vi "test.ingest_containerized.vi"   [LabVIEW 2020]
uses:
  datasources/dataset/dataset.lvclass
  81c5314d-0c17-4e40-9591-806fc92e59be.vi
  Nominal Client/Nominal Client.lvclass
  40e2c779-94f0-4ff6-913c-6196809b7e71.vi
  datasources/source/source.lvclass
  datasources/target/target.lvclass
  nominal types/channelConfig/channelConfig.lvclass
  Nominal Client/ingest_containerized.vi
  datasources/source/create_s3.vi
  datasources/source/create_gcs.vi
  datasources/target/create_from_existing.vi
  datasources/target/create_new.vi
  nominal types/properties/properties.lvclass
  datasources/gcs/gcs.lvclass
  C:/code/labview-client/lv_src/Nominal Client/datasources/source/source.lvclass
  C:/code/labview-client/lv_src/Nominal Client/datasources/payload/payload.lvclass
  C:/code/labview-client/lv_src/Nominal Client/datasources/gcs/gcs.lvclass
  datasources/s3/s3.lvclass
  C:/code/labview-client/lv_src/Nominal Client/datasources/s3/s3.lvclass
types:
  T1 = cluster{"dataset":refnum<class "dataset.lvclass">, "channelConfig":refnum<class "channelConfig.lvclass">}
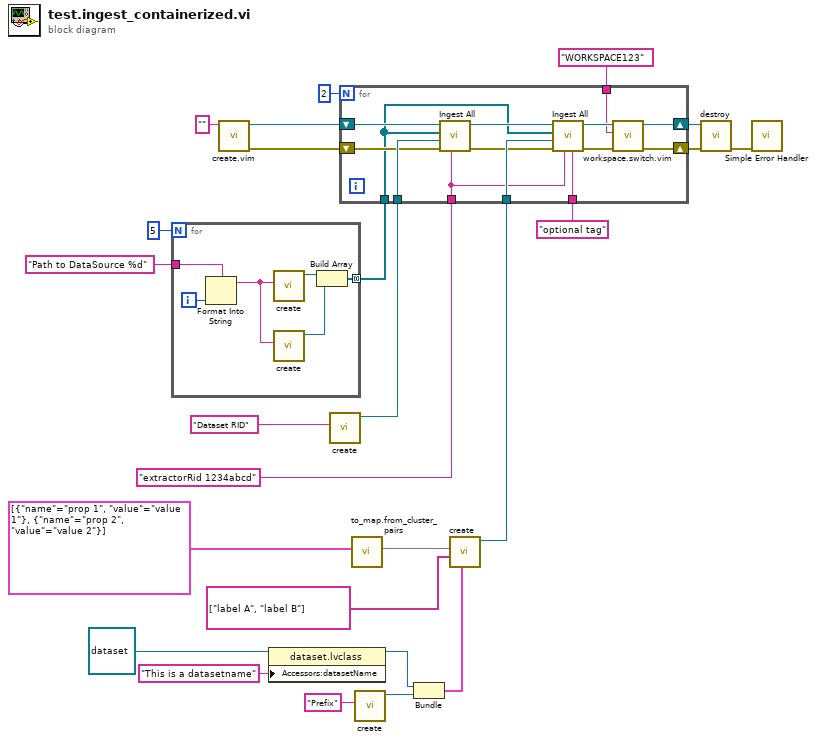
[diagram p0: block diagram]
diagram:
  n1 = for {
    N: 5 -> [_]
    tunnel: "Path to DataSource %d" ("Path") -> [w30]
    tunnel: [w26] -> w7 mode=concatenating
    i -> [w29]
    n2 = Format Into String(format string=w30, w29) -> (resulting string=w31:string)  [unwired: 2 in, 1 out]
    n3 = call-poly "create.vi"("Path"=w31) -> ("source"=w28:refnum<class "gcs.lvclass">)  [unwired: 10 in]
    n4 = call-poly "create.vi"("Path"=w31) -> ("source"=w27:refnum<class "s3.lvclass">)  [unwired: 10 in]
    n5 = Build Array(w28, w27) -> (w26:refnum<class "source.lvclass">[])
  }
  n6 = call "create.vim"("API Token (string or path)"="") -> ("error out"=w21:errorcluster, "Nominal Client"=w22:refnum<class "Nominal Client.lvclass">)  [unwired: 9 in]
  n7 = property class="dataset.lvclass"(reference=refnum<class "dataset.lvclass"> refnum ("dataset"), "Accessors:datasetName"="This is a datasetname" ("datasetName")) -> (reference out=w17:refnum<class "dataset.lvclass">)  [unwired: 1 in, 1 out]
  n8 = call-poly "create.vi"("dataset RID"="Dataset RID" ("RID")) -> ("Existing Target"=w14:refnum<class "target.lvclass">)  [unwired: 10 in]
  n9 = call "to_map.from_cluster_pairs.vi"("properties (cluster pairs)"=cluster{"name":string, "value":string}[] [{"name"="prop 1", "value"="value 1"}, {"name"="prop 2", "value"="value 2"}] ("properties")) -> ("properties (map)"=w1:map{string, string})  [unwired: 10 in]
  n10 = call "create.vi"("prefixTreeDelimiter"="Prefix") -> ("channelConfig"=w10:refnum<class "channelConfig.lvclass">)  [unwired: 10 in]
  n11 = Bundle("dataset"=w17, "channelConfig"=w10) -> (w13:T1)  [unwired: 1 in]
  n12 = call-poly "create.vi"("Optional"=w13, "Labels"=string[] ["label A", "label B"] ("labels"), "Properties"=w1) -> ("New Target"=w12:refnum<class "target.lvclass">)  [unwired: 8 in]
  n13 = for {
    N: 2 -> [_]
    tunnel: w14 -> [w45]
    tunnel: w7 -> [w34]
    tunnel: w12 -> [w44]
    shift-right: [w37] -> w23
    shift-left: w21 -> [w41]
    shift-right: [w36] -> w25
    shift-left: w22 -> [w40]
    tunnel: "WORKSPACE123" ("RID") -> [w35]
    tunnel: "extractorRid 1234abcd" ("RID") -> [w33]
    tunnel: "optional tag" ("RID") -> [w32]
    n14 = call-poly "Ingest All.vi"("extractorRid"=w33, "error in"=w41, "Target"=w45, "sources"=w34, "Nominal Client in"=w40) -> ("error out"=w42:errorcluster, "Nominal Client out"=w43:refnum<class "Nominal Client.lvclass">)  [unwired: 3 in, 2 out]
    n15 = call-poly "Ingest All.vi"("tag"=w32, "extractorRid"=w33, "error in"=w42, "Target"=w44, "sources"=w34, "Nominal Client in"=w43) -> ("error out"=w38:errorcluster, "Nominal Client out"=w39:refnum<class "Nominal Client.lvclass">)  [unwired: 2 in, 2 out]
    n16 = call "workspace.switch.vim"("error in"=w38, "Workspace RID (string or path)"=w35, "Nominal Client in"=w39) -> ("error out"=w37:errorcluster, "Nominal Client out"=w36:refnum<class "Nominal Client.lvclass">)  [unwired: 7 in]
  }
  n17 = call "destroy.vi"("error in"=w23, "Nominal Client"=w25) -> ("error out"=w16:errorcluster)  [unwired: 9 in]
  n18 = call <vilib>:"Simple Error Handler.vi"("error in (no error)"=w16) -> ()  [unwired: 4 in, 5 out]
